vi "Update Core.vi"(8 "error in (no error)":cluster{"状态":bool, "代码":i32, "源":string} caption="错误输入（无错误）", 11 "水位控制器输入":refnum<class "Timed Loop Actor.lvclass">) -> (0 "error out":cluster{"状态":bool, "代码":i32, "源":string} caption="错误输出", 3 "水位控制器输出":refnum<class "Timed Loop Actor.lvclass">)   [LabVIEW 2013, in "Timed Loop Actor.lvlib" / "Timed Loop Actor.lvclass"]
doc: "该VI指定每次循环执行时，由定时循环控制器执行的操作。如需添加待执行的操作，可对子类中的相应VI进行重写，但添加的操作必须在“轮询速率”设定的时间之内执行完毕。子类中只能添加执行时间确定的功能（比如，不能包含异步函数以及依赖于UI线程的操作）。按设计，定时循环控制器类在部署至实时系统时提供确定性可重复的操作，如代码中包含非确定性的部分，可能导致奇怪而难以调试的系统故障。"
uses:
  Timed Loop Actor.lvclass
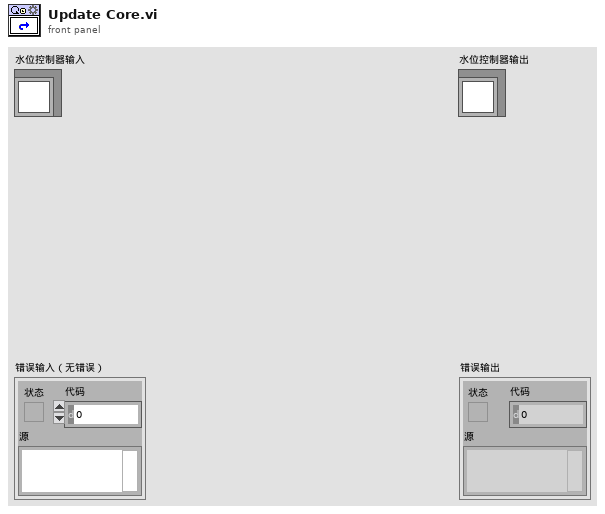
[diagram p1: front panel]
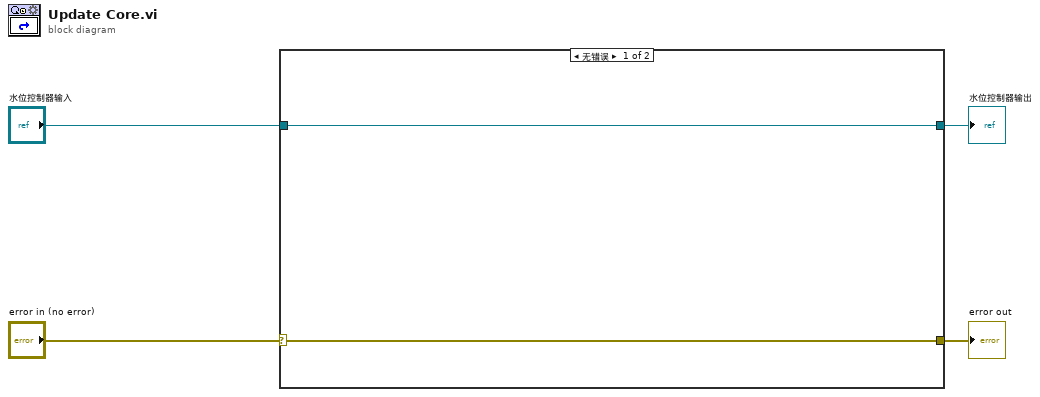
[diagram p0: block diagram]
diagram:
  n1 = case shown="无错误" "error in (no error)" {
    selector: "error in (no error)" -> [w5 w8]
    tunnel: [w5 w8] -> w3
    tunnel: [w6 w7] -> w1
    tunnel: "水位控制器输入" -> [w6 w7]
    frame No Error {
    }
    frame Error {
    }
  }
  "error out" <- w3
  "水位控制器输出" <- w1
